vi "Stop Core.vi"(10 "final error code":i32, 11 "System Actor in":refnum<class "System Actor.lvclass">) -> (3 "System Actor out":refnum<class "System Actor.lvclass">)   [LabVIEW 2014, in "Robot Actor Framework.lvlib" / "System Actor.lvlib" / "System Actor.lvclass"]
doc: "(<B>Filename</B>: Actor Framework.lvlib:Actor.lvclass:Stop Core.vi)\n\nDefines what the actor does before it stops. Use the <B>final error code</B> input to determine whether the actor shut down in response to an error.\n\nBy default, this method does nothing. A descendant class may override it to define behavior, such as shutting down any processes the actor initiated in its override of the Actor Core method."
uses:
  System Actor.lvclass
  System Actor.lvclass/System Actor.ctl
  <vilib>/ActorFramework/Stop Msg/Stop Msg.lvclass/Stop Msg.ctl
  <vilib>/ActorFramework/Message Enqueuer/Message Enqueuer.lvclass/Message Enqueuer.ctl
  <vilib>/ActorFramework/Stop Msg/Send Emergency Stop.vi
  <vilib>/ActorFramework/Stop Msg/Send Normal Stop.vi
  <vilib>/ActorFramework/Message Enqueuer/Enqueue Critical.vi
  <vilib>/ActorFramework/Message Enqueuer/Enqueue.vi
  <vilib>/ActorFramework/Message Priority Queue/Priority Enqueue.vi
  <vilib>/ActorFramework/Stop Msg/Stop Msg.lvclass
  <vilib>/ActorFramework/Actor/Actor.lvclass
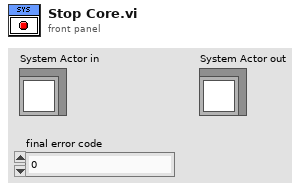
[diagram p1: front panel]
types:
  T1 = enum16{"Critical", "Error", "Warning", "Informational", "Debug"}
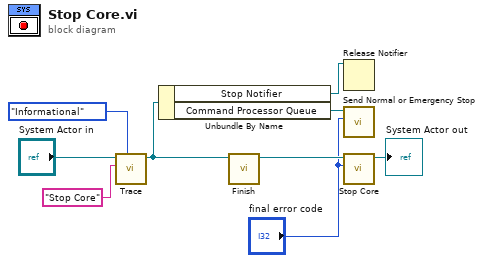
[diagram p0: block diagram]
diagram:
  n1 = call-dynamic "Trace.vi"("Trace Level"=T1."Informational", "System Action"="Stop Core" ("Trace Message"), "System Actor in"="System Actor in") -> ("System Actor out"=w2:refnum<class "System Actor.lvclass">)  [unwired: 7 in, 1 out]
  n2 = Unbundle By Name(w2) -> ("Stop Notifier"=w7:refnum<notifier>, "Command Processor Queue"=w6:refnum<class "Message Enqueuer.lvclass">)
  n3 = call-dynamic "Finish.vi"("System Actor in"=w2) -> ("System Actor out"=w8:refnum<class "System Actor.lvclass">)  [unwired: 9 in, 1 out]
  n4 = Release Notifier(notifier=w7) -> ()  [unwired: 2 in, 3 out]
  n5 = call <vilib>:"Send Normal or Emergency Stop.vi"("final error code"="final error code", "Message Enqueuer"=w6) -> ()  [unwired: 9 in, 1 out]
  n6 = call-parent "Stop Core.vi"("final error code"="final error code", "Actor in"=w8) -> ("Actor out"=→"System Actor out":refnum<class "System Actor.lvclass">)  [unwired: 9 in]
